vi "PicoScope5000aGetTimebase2.vi"(4 "Number of Samples":u32, 6 "Memory Segment":u32, 7 "Acquisition Settings":T2={"preTriggerSamples"=0, "postTriggerSamples"=1000, "timebase"=2} {"postTriggerSamples" format="%_6p"; "preTriggerSamples" format="%_6p"}, 10 "handle in":i16, 11 "error in (no error)":errorcluster) -> (2 "handle out":i16, 3 "error out":errorcluster, 5 "Properties Panel":T1 {"Max Total Capture Time Available (sec)" format="%.3p"; "Sample Frequency" format="%.3p"; "Sample Rate" format="%.3p"; "Max Samples Available" format="%.3p"; "Total Capture Time (sec)" format="%.3p"})   [LabVIEW 2010]
uses:
  ps5000a.dll
  shared/Acquisition Settings.ctl
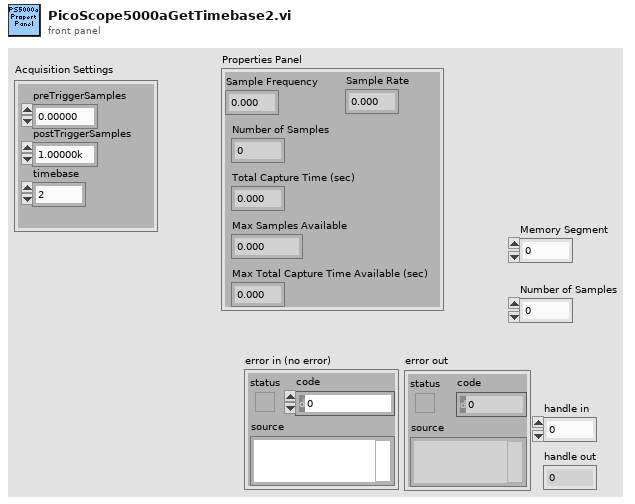
[diagram p1: front panel]
types:
  T1 = cluster{"Sample Frequency":sgl, "Sample Rate":sgl, "Max Samples Available":i32, "Number of Samples":u32, "Total Capture Time (sec) ":sgl, "Max Total Capture Time Available (sec)":sgl}
  T2 = typedef "Acquisition Settings.ctl" = cluster{"preTriggerSamples":u64, "postTriggerSamples":u64, "timebase":u32}
  T3 = cluster{sgl, sgl, "maxSamples":i32, "Number of Samples":u32, sgl, sgl}
  T4 = cluster{"status":bool, "code":u32, "source":string}
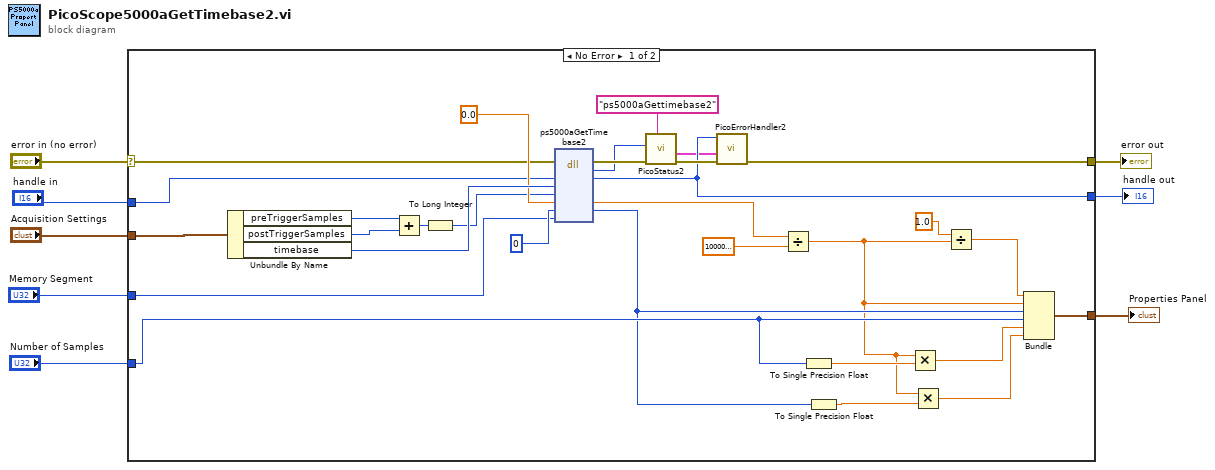
[diagram p0: block diagram]
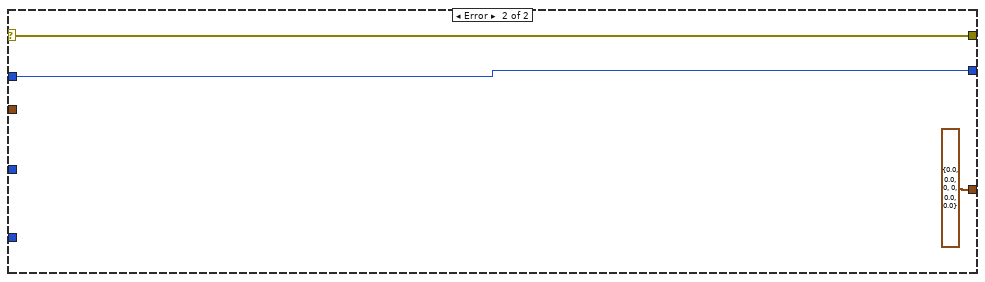
[diagram p2: hidden frame]
diagram:
  n1 = case shown="No Error" "error in (no error)" {
    selector: "error in (no error)" -> [w9 w41]
    tunnel: [w15 w41] -> w8
    tunnel: [w13 w40] -> w7
    tunnel: "Memory Segment" -> [w29 _]
    tunnel: "Number of Samples" -> [w24 _]
    tunnel: "handle in" -> [w28 w40]
    tunnel: "Acquisition Settings" -> [w27 _]
    tunnel: [w20 T3 {0.0, 0.0, "maxSamples"=0, "Number of Samples"=0, 0.0, 0.0}] -> w1
    frame No Error {
      n2 = Unbundle By Name(w27) -> ("preTriggerSamples"=w33:u64, "postTriggerSamples"=w34:u64, "timebase"=w35:u32)
      n3 = Add(x=w33, y=w34) -> (x+y=w11:u64)
      n4 = To Long Integer(number=w11) -> (32bit integer=w12:i32)
      n5 = dll-call lib="ps5000a.dll" fn="ps5000aGetTimebase2"(error in=w9, "handle"=w28, "timebase"=w35, "noSamples"=w12, "timeIntervalNanoseconds"=sgl 0.0, "maxSamples"=0, "segmentIndex"=w29) -> (error out=w36:errorcluster, "PICO_STATUS"=w14:u32, "handle"=w13:i16, "timeIntervalNanoseconds"=w37:sgl, "maxSamples"=w22:i32)  [unwired: 5 in, 1 out]
      n6 = call "PicoStatus2.vi"("PICO source"="ps5000aGettimebase2" ("source"), "Error in"=w36, "PICO STATUS"=w14) -> ("error out"=w16:errorcluster, "PICO_STATUS out"=w10:T4)  [unwired: 5 in]
      n7 = call "PicoErrorHandler2.vi"("error in (no error)"=w16, "PICO_STATUS in"=w10, "handle In"=w13) -> ("error out"=w15:errorcluster)  [unwired: 8 in]
      n8 = Divide(x=w37, y=sgl 1000000000.0) -> (x/y=w19:sgl)
      n9 = To Single Precision Float(number=w24) -> (single precision float=w26:sgl)
      n10 = To Single Precision Float(number=w22) -> (single precision float=w23:sgl)
      n11 = Multiply(x=w19, y=w26) -> (x*y=w25:sgl)
      n12 = Multiply(x=w19, y=w23) -> (x*y=w21:sgl)
      n13 = Divide(x=sgl 1.0, y=w19) -> (x/y=w17:sgl)
      n14 = Bundle(w17, w19, "maxSamples"=w22, "Number of Samples"=w24, w25, w21) -> (w20:T3)  [unwired: 1 in]
    }
    frame Error {
    }
  }
  "error out" <- w8
  "handle out" <- w7
  "Properties Panel" <- w1
